vi "MakeEyeBMP.vi"(0 "Choose Directory":path) -> ()   [LabVIEW 2022 SP3]
uses:
  <vilib>/Analysis/4window.llb/Chebyshev Window (DBL).vi
  <vilib>/Analysis/NI_AALPro.lvlib
panel:
  in  "stripped path":path
  in  "Header format":u16(ring) items=["Riverside Format", "Ron Linear", "GE Bin"]
  out "max dB value":dbl
  in  "dB ref":dbl=98.7
  in  "Relative dB Scale":u16(ring) items=["Each Image", "Bit depth", "Choose dB Value"]
  in  "# rings":i32=1
  in  "Fix dB Range?":bool
  in  "Parse":u16=1
  in  "Filter Prams":T1={"low cutoff"=5, "order"=81, "high cutoff"=35}
  in  "Type of Mean":u16(ring)=3 items=["Mean from lines", "Mean just lines", "Poly Mean", "No mean", "Filter"]
  in  "Flip?":bool=TRUE
  in  "Compress":bool
  in  "Y scale":dbl=1.0
  in  "X scale":dbl=1.0
  in  "file ext":string="*.eye"
  out "Current Image":string
  out "Numeric":i32
  out "Array":dbl[](array[numeric])
  in  "Save Data":bool
  in  "Use Selected Files":bool
  in  "Listbox":i32[](listbox)
  out "Scale factors":dbl[](array[numeric])
  out "BMP to be":dbl[][](graph)
  # "Slect a batch of eye files and the will be saved as BMP 24 bit RGB. They will be converted to a 1to1 aspect ratio and the batch will be scaled to reflect absolute voltage levels. Data is log compressed. May want to adjust Z scale to improve contrast."
  # "Scale in mm"
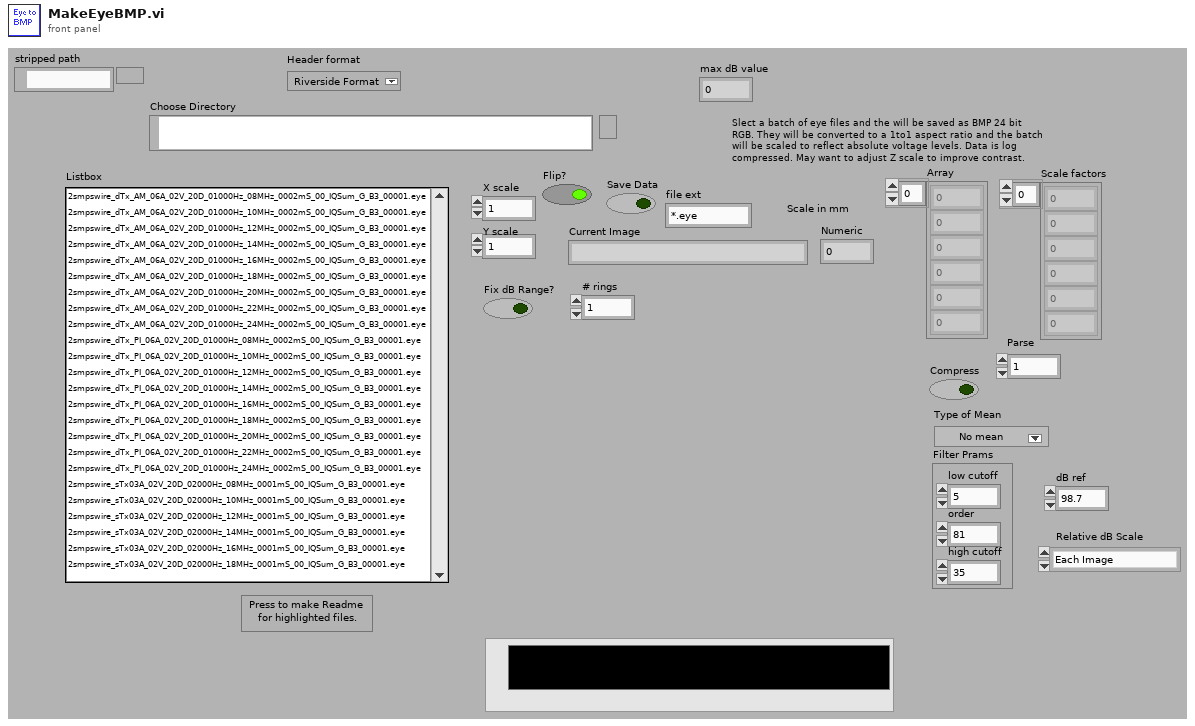
[diagram p1: front panel]
types:
  T1 = cluster{"low cutoff":i32, "order":i32, "high cutoff":i32}
  T2 = typedef "Header.ctl" = cluster{"header info":cluster{"Header":string, "Head length":i16}, "A/D info":cluster{"# rf points per line":u16, "# lines per scan":u16, "sample rate MHz":u16, "# A/D bits":i16, "# bytes per A/D":u16, "TGC Flag":u16, "A/D Type":string}, "Tranducer Info":cluster{"bandwidth":sgl, "center freq":sgl, "start freq":sgl, "ID":i32}, "Scan Info":cluster{"delay":sgl, "pivot distance":sgl, "sector scan angle":sgl, "operator":string, "Scan Mode":string, "location":string}, "Time/Date Info":cluster{"date":string, "time":string}, "RF Info":cluster{"RF file name":string, "RF file att":string, "RF cal file name":string, "RF cal file att":string}, "Patient Info":cluster{"ID":string, "extended ID":string, "age":u16, "sex":string, "previously\nscanned":string, "PSA":sgl, "LOS":u8, "Ethnicty 2":u8, "Race":u8}, "Tissue Type":cluster{"organ":i16, "disease type":i16, "disease location":i16, "IQ_pts":u16, "RcvBuffer":u8, "RcvFrame":u16, "IQBuff":u8, "IQFrame":u16, "IQPage":u8}, "Votage scaling":cluster{"Digitizer (dB)":sgl, "Gain (dB)":sgl, "Atten (dB)":sgl}, "Comment":string, "Misc Info":cluster{"avg num":u16, "c speed":i16, "Div By or SF zones":i16, "XMIT CHS":u8, "RCV CHS":u8, "Xmit angle":sgl}, "Therapy Parameters":cluster{"Theraputic Freq (MHz)":sgl, "Time on (s)":sgl, "Therapy amplitude (mV)":sgl, "Lines Before":u16, "Lines After":u16}, "Scan Settings":cluster{"Energy (uJ or V)":u8, "Damp (Ohm) or Fc":u8, "HP Filt (KHz)":u8, "LP Filt (MHz)":u8, "Gain (db)":u8, "prf (kHz)":sgl, "Distance between\nscan lines (um)":u16, "Distance between\nscan planes (um)":u16, "Scan line gap (um)":sgl, "Scan plane gap (um)":sgl}, "Compression Parameters":cluster{"F1 (MHz)":sgl, "F2 (MHz)":sgl, "% taper":sgl, "duration":sgl}, "Patient Info Xtra":cluster{"First Name":string, "Last Name":string, "Notes":string}, "ROI Box":u16[]}
  T3 = cluster{"Font Name:":string, "Size":i16, "Strikeout?":bool, "Italic?":bool, "Underline?":bool, "Outline?":bool, "Shadow?":bool, "Bold?":bool}
  T4 = cluster{"left":i16, "top":i16, "right":i16, "bottom":i16}
  T5 = enum16{"User-specified Font", "Application Font", "System Font", "Dialog Font"}
  T6 = enum16{"None", "Stacked", "Clockwise", "Counterclockwise"}
  T7 = cluster{"F1 (MHz)":sgl, "F2 (MHz)":sgl, "% taper":sgl, "duration":sgl}
  T8 = cluster{cluster{dbl, dbl}, dbl, dbl, "delay":sgl, "delay":sgl, dbl, dbl}
  T9 = typedef "imagedata.ctl" = cluster{"image type":i32, "image depth":i32, "image":u8[], "mask":u8[], "colors":u32[], "Rectangle":cluster{"left":i16, "top":i16, "right":i16, "bottom":i16}}
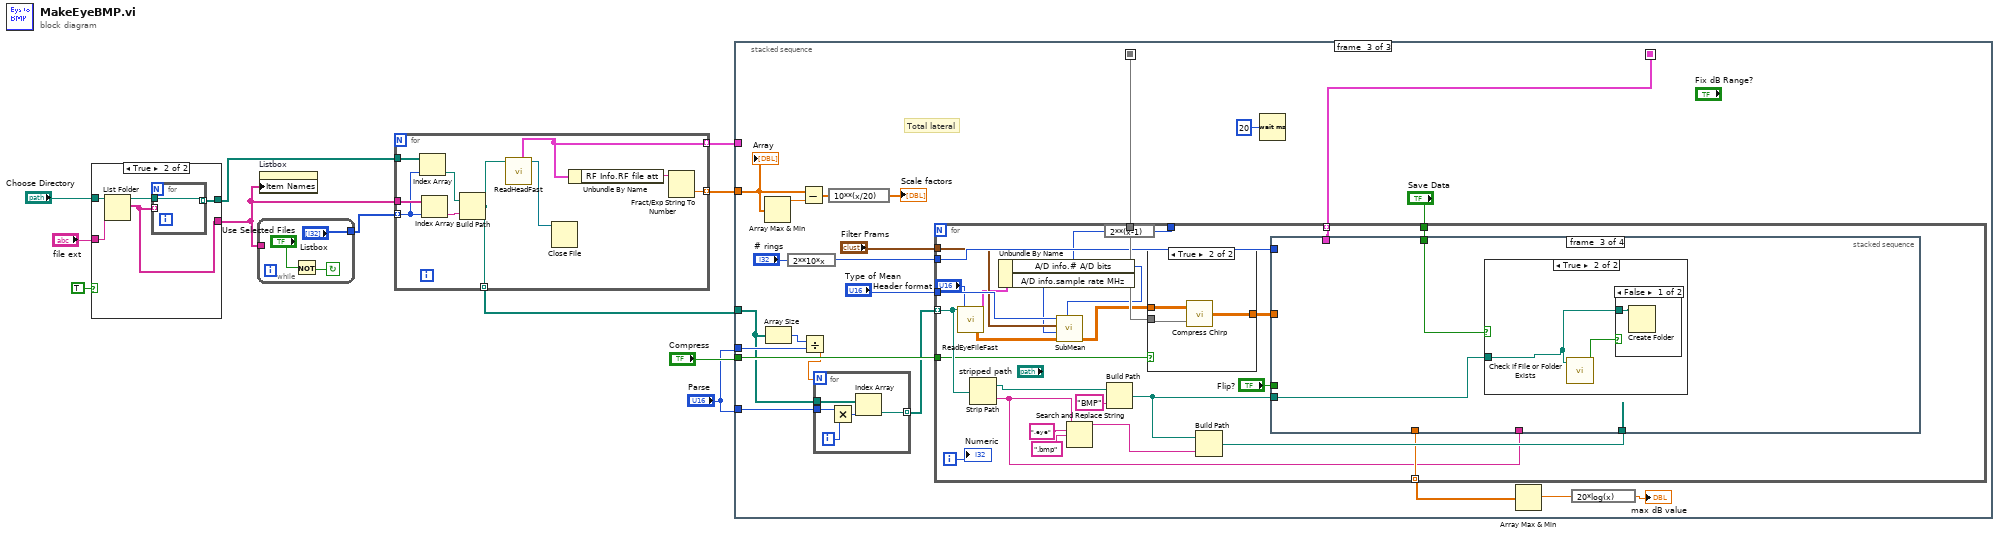
[diagram p0: block diagram]
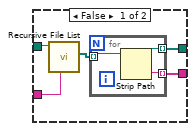
[diagram p2: hidden frame]
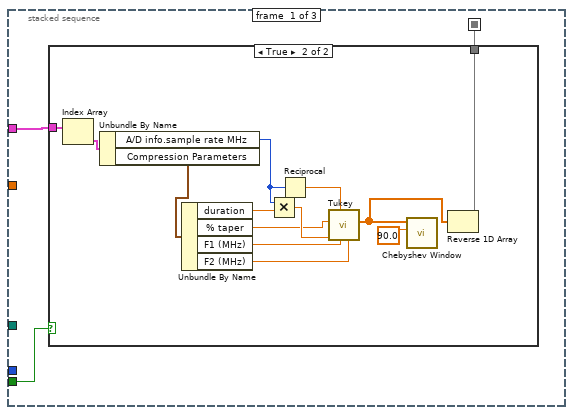
[diagram p3: hidden frame]
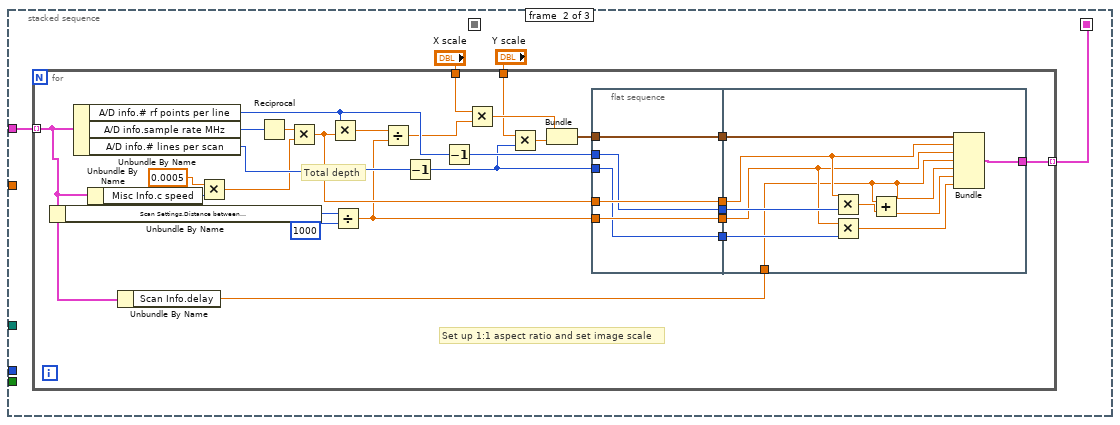
[diagram p5: hidden frame]
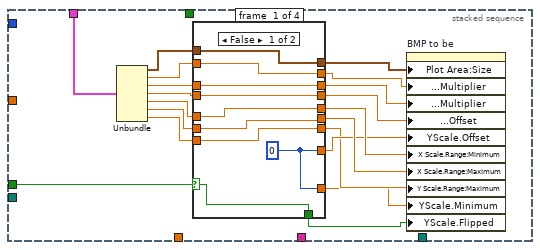
[diagram p7: hidden frame]
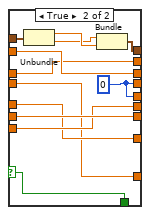
[diagram p8: hidden frame]
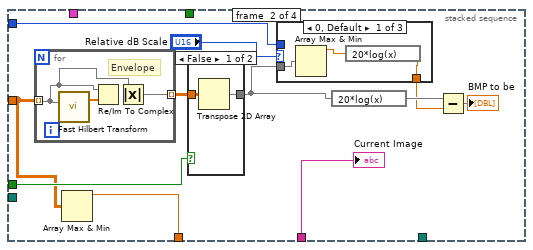
[diagram p9: hidden frame]
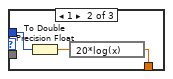
[diagram p10: hidden frame]
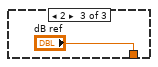
[diagram p11: hidden frame]
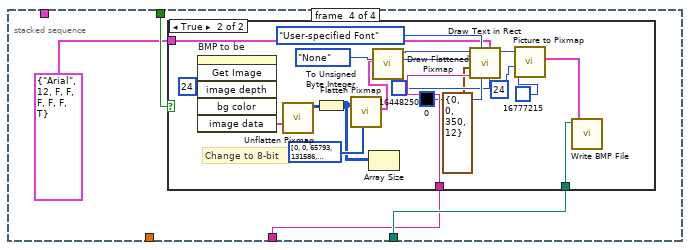
[diagram p15: hidden frame]
diagram:
  n1 = case shown="True" TRUE {
    tunnel: [w13 w22] -> w9
    tunnel: "Choose Directory" -> [w16 w24]
    tunnel: [w14 w20] -> w5
    tunnel: "file ext" -> [w12 w23]
    frame False {
      n2 = call <vilib>:"Recursive File List.vi"("pattern"=w12, "Folder Path"=w16) -> ("All Files in Dir"=w15:path[])  [unwired: 5 in, 4 out]
      n3 = for {
        tunnel: w15 -> [w19] mode=indexing
        tunnel: [w18] -> w14 mode=indexing
        tunnel: [w17] -> w13 mode=indexing
        n4 = Strip Path(path=w19) -> (stripped path=w18:path, name=w17:string)
      }
    }
    frame True {
      n5 = List Folder(path=w24, pattern=w23) -> (path out=w21:path, filenames=w22:string[])  [unwired: 1 in, 3 out]
      n6 = for {
        tunnel: w21 -> [w25]
        tunnel: w22 -> [_] mode=indexing
        tunnel: [w25] -> w20 mode=indexing
      }
    }
  }
  n7 = while {
    tunnel: ["Listbox"] -> w8
    tunnel: w9 -> [_]
    stop <- w28 continue-if-true
    n8 = Not(x="Use Selected Files") -> (.not. x?=w28:bool)
  }
  n9 = property on="Listbox" class="LstBox (strict)"("Item Names"=w9) -> ()  [unwired: 2 in, 2 out]
  n10 = for {
    tunnel: [w37] -> w10 mode=indexing
    tunnel: [w33] -> w11 mode=indexing
    tunnel: w9 -> [w36]
    tunnel: w8 -> [w29] mode=indexing
    tunnel: [w34] -> w7 mode=indexing
    tunnel: w5 -> [w31]
    n11 = Index Array(array=w31, index=w29) -> (element=w30:path)
    n12 = Index Array(array=w36, index=w29) -> (element=w35:string)
    n13 = Build Path(base path=w30, name or relative path=w35) -> (appended path=w34:path)
    n14 = call "ReadHeadFast.vi"("new file path"=w34) -> ("refnum out"=w32:refnum<file>, "Header In"=w33:T2)  [unwired: 7 in, 2 out]
    n15 = Close File(refnum=w32) -> ()  [unwired: 1 in, 2 out]
    n16 = Unbundle By Name(w33) -> ("RF Info.RF file att"=w38:string)
    n17 = Fract/Exp String To Number(string=w38) -> (number=w37:dbl)  [unwired: 4 out]
  }
  n18 = stacked-sequence {
    seq-local: [_ w57 _] -> [_ _ w119]
    seq-local: [w40 _ _] -> [_ _ w117]
    tunnel: w11 -> [w41 w58 _]
    tunnel: w10 -> [_ _ w123]
    tunnel: w7 -> [_ _ w110]
    tunnel: "Compress" -> [w39 _ w118]
    tunnel: "Parse" -> [_ _ w112]
    tunnel: "Parse" -> [_ _ w109]
    frame #0 {
      n19 = case shown="True" w39 {
        tunnel: w41 -> [_ w46]
        tunnel: [_ w44] -> w40
        frame False {
        }
        frame True {
          n20 = Index Array(array=w46) -> (element=w45:T2)  [unwired: 1 in]
          n21 = Unbundle By Name(w45) -> ("A/D info.sample rate MHz"=w47:u16, "Compression Parameters"=w42:T7)
          n22 = Unbundle By Name(w42) -> ("duration"=w54:sgl, "% taper"=w49:sgl, "F1 (MHz)"=w53:sgl, "F2 (MHz)"=w52:sgl)
          n23 = Multiply(x=w47, y=w54) -> (x*y=w50:sgl)
          n24 = Reciprocal(x=w47) -> (1/x=w51:dbl)
          n25 = call "Tukey.vi"("f2 (MHz)"=w52, "f1 (MHz)"=w53, "Samp Rate (mics)"=w51, "Pts"=w50, "Tukey"=w49) -> ("Tukey Chirp"=w43:dbl[])  [unwired: 2 in, 4 out]
          n26 = call-poly <vilib>:"Chebyshev Window.vi"("lobe ratio (dB)"=90.0, "X"=w43) -> ()  [unwired: 10 out]
          n27 = Reverse 1D Array(array=w43) -> (reversed array=w44:dbl[])
        }
      }
    }
    frame #1 {
      n28 = for {
        tunnel: w58 -> [w59] mode=indexing
        tunnel: [w67] -> w57 mode=indexing
        tunnel: "X scale" -> [w61]
        tunnel: "Y scale" -> [w60]
        # "Set up 1:1 aspect ratio and set image scale"
        # "Total depth"
        n29 = Unbundle By Name(w59) -> ("Scan Settings.Distance between\nscan lines (um)"=w74:u16)
        n30 = Unbundle By Name(w59) -> ("A/D info.# rf points per line"=w77:u16, "A/D info.sample rate MHz"=w79:u16, "A/D info.# lines per scan"=w76:u16)
        n31 = Unbundle By Name(w59) -> ("Misc Info.c speed"=w73:i16)
        n32 = Unbundle By Name(w59) -> ("Scan Info.delay"=w69:sgl)
        n33 = Multiply(x=0.0005, y=w73) -> (x*y=w71:dbl)
        n34 = Reciprocal(x=w79) -> (1/x=w80:dbl)
        n35 = Multiply(x=w80, y=w71) -> (x*y=w70:dbl)
        n36 = Multiply(x=w77, y=w70) -> (x*y=w78:dbl)
        n37 = Divide(x=w74, y=1000) -> (x/y=w68:dbl)
        n38 = Divide(x=w78, y=w68) -> (x/y=w65:dbl)
        n39 = Decrement(x=w76) -> (x-1=w63:u16)
        n40 = Decrement(x=w77) -> (x-1=w75:u16)
        n41 = Multiply(x=w61, y=w65) -> (x*y=w64:dbl)
        n42 = Multiply(x=w60, y=w63) -> (x*y=w62:dbl)
        n43 = Bundle(w64, w62) -> (w66:cluster{dbl, dbl})  [unwired: 1 out]
        n44 = flat-sequence {
          tunnel: w75 -> [w88]
          tunnel: w63 -> [w89]
          tunnel: w66 -> [w87]
          tunnel: [w91] -> w86
          tunnel: w70 -> [w91]
          tunnel: [w90] -> w85
          tunnel: w68 -> [w90]
          tunnel: [w89] -> w84
          tunnel: [w88] -> w83
          tunnel: [w87] -> w82
          tunnel: w86 -> [w97]
          tunnel: w69 -> [w95]
          tunnel: w85 -> [w96]
          tunnel: w84 -> [w101]
          tunnel: w83 -> [w100]
          tunnel: w82 -> [w98]
          tunnel: [w92] -> w67
          frame #0 {
          }
          frame #1 {
            n45 = Multiply(x=w97, y=w100) -> (x*y=w99:dbl)
            n46 = Multiply(x=w96, y=w101) -> (x*y=w93:dbl)
            n47 = Add(x=w95, y=w99) -> (x+y=w94:dbl)
            n48 = Bundle(w98, w97, w96, "delay"=w95, "delay"=w95, w94, w93) -> (w92:T8)  [unwired: 1 out]
          }
        }
      }
    }
    frame #2 {
      # "Total lateral"
      n49 = Array Max & Min(array=w123) -> (max value=w122:dbl)  [unwired: 3 out]
      n50 = Array Size(array=w110) -> (size(s)=w113:i32)
      n51 = expression code="2**10*x"("# rings") -> (w115:i32)
      n52 = Subtract(x=w123, y=w122) -> (x-y=w121:dbl[])
      n53 = Divide(x=w113, y=w112) -> (x/y=w111:dbl)
      n54 = for {
        N: w111 -> [_]
        tunnel: w110 -> [w127]
        tunnel: w109 -> [w126]
        tunnel: [w125] -> w108 mode=indexing
        i -> [w128]
        n55 = Multiply(x=w126, y=w128) -> (x*y=w124:i32)
        n56 = Index Array(array=w127, index=w124) -> (element=w125:path)
      }
      n57 = expression code="10**(x/20)"(w121) -> (→"Scale factors":dbl[])
      n58 = for {
        tunnel: w108 -> [w155] mode=indexing
        tunnel: "Save Data" -> [w151]
        tunnel: w119 -> [w147] mode=indexing
        tunnel: "Type of Mean" -> [w146]
        tunnel: w118 -> [w145]
        tunnel: w117 -> [w144]
        tunnel: w115 -> [w139]
        tunnel: [w138] -> _
        tunnel: "Filter Prams" -> [w137]
        tunnel: [w133] -> w105 mode=indexing
        i -> [w150]
        n59 = call "ReadEyeFileFast.vi"("new file path"=w155, "Header format"="Header format") -> ("2-D data array"=w142:sgl[][], "Header In"=w136:T2)  [unwired: 16 out]
        n60 = Strip Path(path=w155) -> (stripped path=w129:path, name=w132:string)
        n61 = Unbundle By Name(w136) -> ("A/D info.# A/D bits"=w134:i16, "A/D info.sample rate MHz"=w135:u16)
        n62 = call "SubMean.vi"("Bit Depth"=w134, "Scan Data In"=w142, "Samp Rate (MHz)"=w135, "Filter Prams"=w137, "Type of Mean"=w146) -> ("Array"=w143:dbl[][])  [unwired: 1 in, 2 out]
        n63 = Search and Replace String(input string=w132, search string=".eye", replace string=".bmp") -> (result string=w148:string)  [unwired: 1 in, 7 out]
        n64 = expression code="2**(x-1)"(w134) -> (w138:i16)
        n65 = Build Path(base path=w129, name or relative path="BMP") -> (appended path=w130:path)
        n66 = case shown="True" w145 {
          tunnel: w143 -> [w156 w159]
          tunnel: [w156 w158] -> w141
          tunnel: w144 -> [_ w157]
          frame False {
          }
          frame True {
            n67 = call "Compress Chirp.vi"("Chirp"=w157, "Array In"=w159) -> ("Array Out"=w158:dbl[][])
          }
        }
        n68 = Build Path(base path=w130, name or relative path=w148) -> (appended path=w152:path)
        n69 = stacked-sequence {
          tunnel: w132 -> [_ w210 _ w230]
          tunnel: w152 -> [_ _ _ w232]
          tunnel: w151 -> [_ _ w224 w231]
          tunnel: w147 -> [w178 _ _ _]
          tunnel: w141 -> [_ w201 _ _]
          tunnel: "Flip?" -> [w162 w208 _ _]
          tunnel: w139 -> [_ w202 _ _]
          tunnel: [_ w200 _ _] -> w133
          tunnel: w130 -> [_ _ w225 _]
          frame #0 {
            n70 = Unbundle(w178) -> (w171:cluster{dbl, dbl}, w172:dbl, w177:dbl, "delay"=w176:sgl, "delay"=w175:sgl, w174:dbl, w173:dbl)
            n71 = case shown="False" w162 {
              selector: w162 -> [w179 w188]
              tunnel: [w187 w199] -> w168
              tunnel: w177 -> [w187 w198]
              tunnel: [w186 w190] -> w167
              tunnel: w176 -> [w186 w189]
              tunnel: [w180 w190] -> w166
              tunnel: w175 -> [w180 w191]
              tunnel: [w182 w196] -> w165
              tunnel: w174 -> [w182 w197]
              tunnel: [w185 w197] -> w163
              tunnel: w173 -> [w185 w196]
              tunnel: [w184 w198] -> w169
              tunnel: w172 -> [w184 w199]
              tunnel: [w183 w192] -> w170
              tunnel: w171 -> [w183 w195]
              tunnel: [w181 w191] -> w164
              tunnel: [w181 w189] -> w161
              tunnel: [w179 w188] -> w160
              frame False {
                w181 = 0
              }
              frame True {
                w190 = 0
                n72 = Unbundle(w195) -> (w194:dbl, w193:dbl)
                n73 = Bundle(w193, w194) -> (w192:cluster{dbl, dbl})  [unwired: 1 in]
              }
            }
            n74 = property on="BMP to be" class="IntGraph (strict)"("Plot Area:Size"=w170, "X Scale.Offset and Multiplier:Multiplier"=w169, "Y Scale.Offset and Multiplier:Multiplier"=w168, "X Scale.Offset and Multiplier:Offset"=w167, "YScale.Offset"=w164, "X Scale.Range:Minimum"=w166, "X Scale.Range:Maximum"=w165, "Y Scale.Range:Maximum"=w163, "YScale.Minimum"=w161, "YScale.Flipped"=w160) -> ()  [unwired: 2 in, 2 out]
          }
          frame #1 {
            n75 = for {
              tunnel: w201 -> [w221] mode=indexing
              tunnel: [w222] -> w209 mode=indexing
              # "Envelope"
              n76 = call <vilib>:"Fast Hilbert Transform.vi"("X"=w221) -> ("Hilbert{X}"=w223:dbl[])  [unwired: 1 out]
              n77 = Re/Im To Complex(1:w223, 2:w221) -> ()  [unwired: 1 out]
              n78 = Absolute Value(x=w221) -> (abs(x)=w222:dbl[])
            }
            n79 = Array Max & Min(array=w201) -> (max value=w200:dbl)  [unwired: 3 out]
            n80 = case shown="False" w208 {
              tunnel: w209 -> [w219 w220]
              tunnel: [w218 w220] -> w205
              frame False {
                n81 = Transpose 2D Array(2D array=w219) -> (transposed array=w218:dbl[][])
              }
              frame True {
              }
            }
            n82 = case shown="0, Default" "Relative dB Scale" {
              tunnel: w205 -> [w213 _ _]
              tunnel: [w211 w215 "dB ref"] -> w204
              tunnel: w202 -> [_ w216 _]
              frame 0, Default {
                n83 = Array Max & Min(array=w213) -> (max value=w212:dbl)  [unwired: 3 out]
                n84 = expression code="20*log(x)"(w212) -> (w211:dbl)
              }
              frame 1 {
                n85 = To Double Precision Float(number=w216) -> (double precision float=w214:dbl)
                n86 = expression code="20*log(x)"(w214) -> (w215:dbl)
              }
              frame 2 {
              }
            }
            n87 = expression code="20*log(x)"(w205) -> (w207:dbl[][])
            n88 = Subtract(x=w207, y=w204) -> (x-y=→"BMP to be":dbl[][])
            "Current Image" <- w210
          }
          frame #2 {
            n89 = case shown="True" w224 {
              tunnel: w225 -> [_ w226]
              frame False {
              }
              frame True {
                n90 = call <vilib>:"Check if File or Folder Exists.vi"("path"=w226) -> ("file or folder exists?"=w227:bool)  [unwired: 8 in, 2 out]
                n91 = case shown="False" w227 {
                  tunnel: w226 -> [w228 _]
                  frame False {
                    n92 = Create Folder(path (use dialog)=w228) -> ()  [unwired: 1 in, 4 out]
                  }
                  frame True {
                  }
                }
              }
            }
          }
          frame #3 {
            n93 = case shown="True" w231 {
              tunnel: w232 -> [_ w249]
              tunnel: w230 -> [_ w245]
              tunnel: T3 {"Font Name:"="Arial", "Size"=12, "Strikeout?"=FALSE, "Italic?"=FALSE, "Underline?"=FALSE, "Outline?"=FALSE, "Shadow?"=FALSE, "Bold?"=TRUE} ("[user-specified font]") -> [_ w234]
              frame False {
              }
              frame True {
                # "Change to 8-bit"
                n94 = invoke on="BMP to be" class="IntGraph (strict)" method="Get Image"("image depth"=24) -> ("image data"=w250:T9)  [unwired: 5 in, 5 out]
                n95 = call <vilib>:"Unflatten Pixmap.vi"("image data"=w250) -> ("24-bit pixmap"=w247:u32[][])  [unwired: 10 out]
                n96 = To Unsigned Byte Integer(number=w247) -> (unsigned 8bit integer=w233:u8[][])
                n97 = call <vilib>:"Flatten Pixmap.vi"("colors"=u32[] [0, 0, 65793, 131586, 197379, 263172, 328965, 394758, 460551, 526344, 592137, 657930, 723723, 789516, 855309, 921102, 986895, 1052688, 1118481, 1184274, 1250067, 1315860, 1381653, 1447446, 1513239, 1579032, 1644825, 1710618, 1776411, 1842204, 1907997, 1973790, 2039583, 2105376, 2171169, 2236962, 2302755, 2368548, 2434341, 2500134, 2565927, 2631720, 2697513, 2763306, 2829099, 2894892, 2960685, 3026478, 3092271, 3158064, 3223857, 3289650, 3355443, 3421236, 3487029, 3552822, 3618615, 3684408, 3750201, 3815994, 3881787, 3947580, 4013373, 4079166, 4144959, 4210752, 4276545, 4342338, 4408131, 4473924, 4539717, 4605510, 4671303, 4737096, 4802889, 4868682, 4934475, 5000268, 5066061, 5131854, 5197647, 5263440, 5329233, 5395026, 5460819, 5526612, 5592405, 5658198, 5723991, 5789784, 5855577, 5921370, 5987163, 6052956, 6118749, 6184542, 6250335, 6316128, 6381921, 6447714, 6513507, 6579300, 6645093, 6710886, 6776679, 6842472, 6908265, 6974058, 7039851, 7105644, 7171437, 7237230, 7303023, 7368816, 7434609, 7500402, 7566195, 7631988, 7697781, 7763574, 7829367, 7895160, 7960953, 8026746, 8092539, 8158332, 8224125, 8289918, 8355711, 8421504, 8487297, 8553090, 8618883, 8684676, 8750469, 8816262, 8882055, 8947848, 9013641, 9079434, 9145227, 9211020, 9276813, 9342606, 9408399, 9474192, 9539985, 9605778, 9671571, 9737364, 9803157, 9868950, 9934743, 10000536, 10066329, 10132122, 10197915, 10263708, 10329501, 10395294, 10461087, 10526880, 10592673, 10658466, 10724259, 10790052, 10855845, 10921638, 10987431, 11053224, 11119017, 11184810, 11250603, 11316396, 11382189, 11447982, 11513775, 11579568, 11645361, 11711154, 11776947, 11842740, 11908533, 11974326, 12040119, 12105912, 12171705, 12237498, 12303291, 12369084, 12434877, 12500670, 12566463, 12632256, 12698049, 12763842, 12829635, 12895428, 12961221, 13027014, 13092807, 13158600, 13224393, 13290186, 13355979, 13421772, 13487565, 13553358, 13619151, 13684944, 13750737, 13816530, 13882323, 13948116, 14013909, 14079702, 14145495, 14211288, 14277081, 14342874, 14408667, 14474460, 14540253, 14606046, 14671839, 14737632, 14803425, 14869218, 14935011, 15000804, 15066597, 15132390, 15198183, 15263976, 15329769, 15395562, 15461355, 15527148, 15592941, 15658734, 15724527, 15790320, 15856113, 15921906, 15987699, 16053492, 16119285, 16185078, 16250871, 16316664, 16382457, 16448250, 16514043, 16579836, 16645629, 16448250] ("Array 2"), "8-bit pixmap"=w233) -> ("image data"=w241:T9)  [unwired: 4 in, 5 out]
                n98 = Array Size(array=w233) -> ()  [unwired: 1 out]
                n99 = call <vilib>:"Draw Flattened Pixmap.vi"("image data"=w241) -> ("new picture"=w246:picture)  [unwired: 8 in]
                n100 = call <vilib>:"Draw Text in Rect.vi"("BG color(transparent)"=u32 16448250, "[user-specified font]"=w234, "text color(black)"=u32 0, "desired font(Application)"=T5."User-specified Font", "text"=w245, "rect"=T4 {"left"=0, "top"=0, "right"=350, "bottom"=12}, "text orientation"=T6."None", "picture"=w246) -> ("new picture"=w244:picture)  [unwired: 3 in]
                n101 = call <vilib>:"Picture to Pixmap.vi"("Background Color"=u32 16777215, "depth"=24, "picture"=w244) -> ("image data"=w240:T9)  [unwired: 7 in, 1 out]
                n102 = call <vilib>:"Write BMP File.vi"("image data"=w240, "path to BMP file"=w249) -> ()  [unwired: 1 in, 9 out]
              }
            }
          }
        }
        "Numeric" <- w150
      }
      n103 = Wait (ms)(milliseconds to wait=u32 20) -> ()  [unwired: 1 out]
      n104 = Array Max & Min(array=w105) -> (max value=w104:dbl)  [unwired: 3 out]
      n105 = expression code="20*log(x)"(w104) -> (→"max dB value":dbl)
      "Array" <- w123
    }
  }
